vi "Drive_Loop_Gyro_Angle.vi"(10 "Yaw Wind":dbl, 11 "Drive Loop Cluster":T1) -> ()   [LabVIEW 2016]
doc: "Help written by FRC Team 836 - The RoboBees\n\nThis VI writes a set gyro angle into the Gyro Data RT FIFO.\n\nThe RT FIFO has to be intialized using the \"Drive_Loop_Initialize_w_Help\" VI."
uses:
  <userlib>/836-libraries/Drive/Drive_Code/Drive_Code_Support/Drive_Code_Bundle.ctl
  <userlib>/836-libraries/Drive/Drive_Code/Drive_Code_Support/Sensor_Cluster.ctl
  <userlib>/836-libraries/Drive/Drive_Code/Drive_Code_Support/Camera_Cluster.ctl
  <userlib>/836-libraries/Drive/Drive_Code/Drive_Code_Support/Drive_Code_Notifier.ctl
  <userlib>/836-libraries/Drive/Drive_Code/Drive_Code_Support/Drive_Code_Command.ctl
  <userlib>/836-libraries/Drive/Drive_Code/Logging_Data.ctl
  <userlib>/836-libraries/Drive/Drive_Code/Drive_Code_Support/Drive_Code_PID_Bundle.ctl
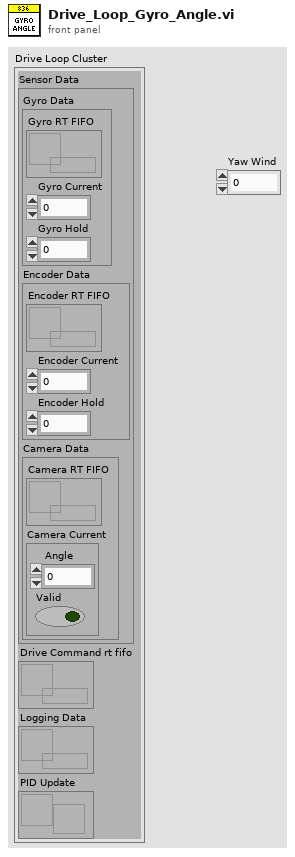
[diagram p1: front panel]
types:
  T1 = typedef "Drive_Code_Bundle.ctl" = cluster{"Sensor Data":T2, "Drive Command rt fifo":refnum<k33>, "Logging Data":refnum<k33>, "PID Update":refnum<notifier>}
  T2 = typedef "Sensor_Cluster.ctl" = cluster{"Gyro Data":cluster{"Gyro RT FIFO":refnum<k33>, "Gyro Current":dbl, "Gyro Hold":dbl}, "Encoder Data":cluster{"Encoder RT FIFO":refnum<k33>, "Encoder Current":dbl, "Encoder Hold":dbl}, "Camera Data":cluster{"Camera RT FIFO":refnum<k33>, "Camera Current":T3}}
  T3 = typedef "Camera_Cluster.ctl" = cluster{" Angle":dbl, "Valid":bool}
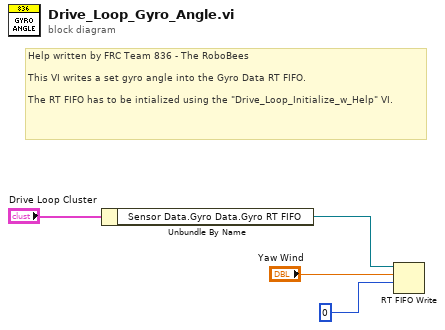
[diagram p0: block diagram]
diagram:
  # "Help written by FRC Team 836 - The RoboBees\n\nThis VI writes a set gyro angle into the Gyro Data RT FIFO.\n\nThe RT FIFO has to be intialized using the \"Drive_Loop_Initialize_w_Help\" VI."
  n1 = Unbundle By Name("Drive Loop Cluster") -> ("Sensor Data.Gyro Data.Gyro RT FIFO"=w4:refnum<k33>)
  n2 = RT FIFO Write(0:w4, 1:"Yaw Wind", 2:0 ("timeout in ms (0)")) -> ()  [unwired: 2 in, 4 out]
